vi "Const-BaudDetect-Array.vi"() -> (0 "DetectArray":cluster{"T0":u8, "T1":u8, "br_selfdef":T1}[](array[cluster]) {"T0" format="%08b"; "T1" format="%08b"; "br_selfdef"."PHSEG2" items=["CAN_BIT_1TQ"=1, "CAN_BIT_2TQ"=2, "CAN_BIT_3TQ"=3, "CAN_BIT_4TQ"=4, "CAN_BIT_5TQ"=5, "CAN_BIT_6TQ"=6, "CAN_BIT_7TQ"=7, "CAN_BIT_8TQ"=8]; "br_selfdef"."PHSEG1" items=["CAN_BIT_1TQ"=1, "CAN_BIT_2TQ"=2, "CAN_BIT_3TQ"=3, "CAN_BIT_4TQ"=4, "CAN_BIT_5TQ"=5, "CAN_BIT_6TQ"=6, "CAN_BIT_7TQ"=7, "CAN_BIT_8TQ"=8]; "br_selfdef"."PRSEG" items=["CAN_BIT_1TQ"=1, "CAN_BIT_2TQ"=2, "CAN_BIT_3TQ"=3, "CAN_BIT_4TQ"=4, "CAN_BIT_5TQ"=5, "CAN_BIT_6TQ"=6, "CAN_BIT_7TQ"=7, "CAN_BIT_8TQ"=8]; "br_selfdef"."PHS2_SEL" items=["由相位缓冲段1时间指定", "可编程"]; "br_selfdef"."SAM" items=["采样一次", "采样三次"]; "br_selfdef"."BRP" items=["1"=1, "2"=2, "3"=3, "4"=4, "5"=5, "6"=6, "7"=7, "8"=8, "9"=9, "10"=10, "11"=11, "12"=12, "13"=13, "14"=14, "15"=15, "16"=16, "17"=17, "18"=18, "19"=19, "20"=20, "21"=21, "22"=22, "23"=23, "24"=24, "25"=25, "26"=26, "27"=27, "28"=28, "29"=29, "30"=30, "31"=31, "32"=32, "33"=33, "34"=34, "35"=35, "36"=36, "37"=37, "38"=38, "39"=39, "40"=40, "41"=41, "42"=42, "43"=43, "44"=44, "45"=45, "46"=46, "47"=47, "48"=48, "49"=49, "50"=50, "51"=51, "52"=52, "53"=53, "54"=54, "55"=55, "56"=56, "57"=57, "58"=58, "59"=59, "60"=60, "61"=61, "62"=62, "63"=63, "64"=64]; "br_selfdef"."SJW" items=["1TQ"=1, "2TQ"=2, "3TQ"=3, "4TQ"=4]; "br_selfdef"."SYN(nouse)" items=["CAN_BIT_1TQ"=1]})   [LabVIEW 2011]
uses:
  Baud rate Self Define.ctl
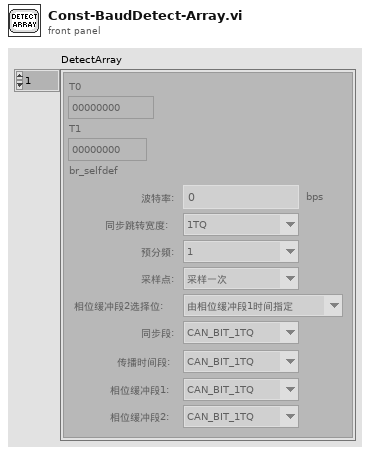
[diagram p1: front panel]
types:
  T1 = typedef "Baud rate Self Define.ctl" = cluster{"BAUD":u32, "SJW":u8, "BRP":u8, "SAM":u8, "PHS2_SEL":u8, "SYN(nouse)":u8, "PRSEG":u8, "PHSEG1":u8, "PHSEG2":u8}
  T2 = cluster{dbl, cluster{"T0":u8, "T1":u8, "br_selfdef":T1}}
  T3 = cluster{dbl, cluster{"T0":u8, "T1":u8, "br_selfdef":T1}}[]
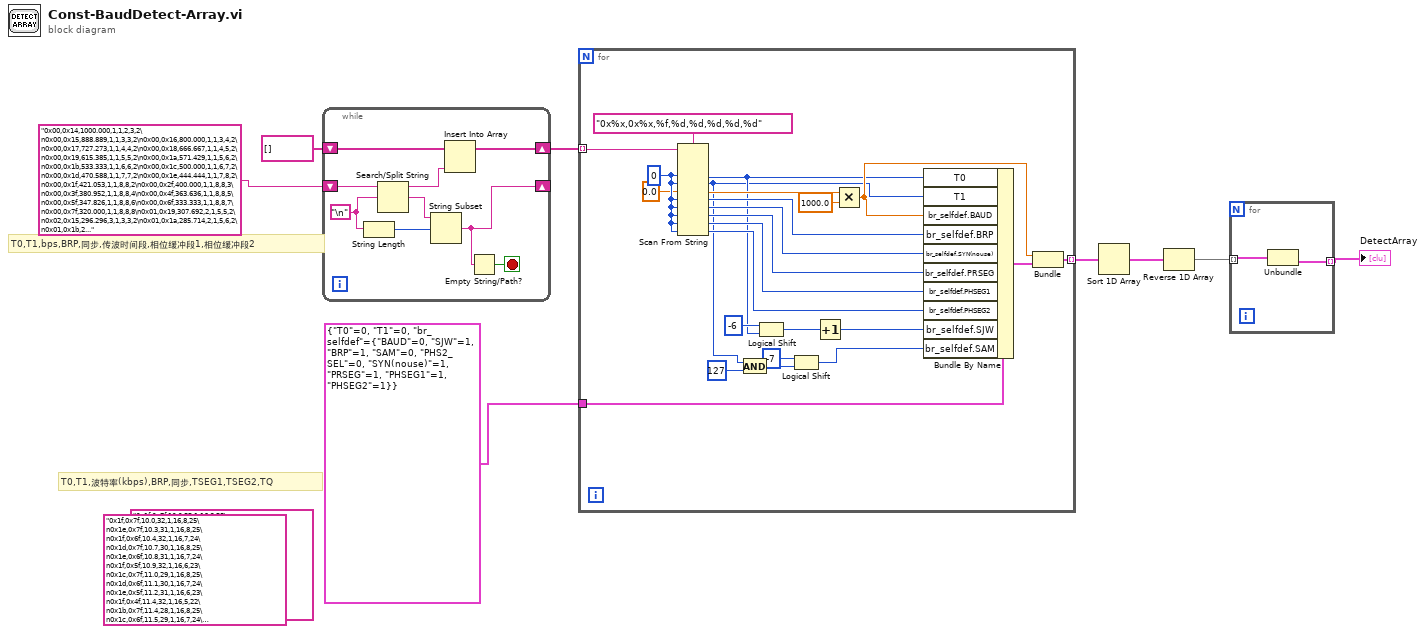
[diagram p0: block diagram]
diagram:
  (unwired) "0x1f,0x7f,10.0,32,1,16,8,25\n0x1e,0x7f,10.3,31,1,16,8,25\n0x1f,0x6f,10.4,32,1,16,7,24\n0x1d,0x7f,10.7,30,1,16,8,25\n0x1e,0x6f,10.8,31,1,16,7,24\n0x1f,0x5f,10.9,32,1,16,6,23\n0x1c,0x7f,11.0,29,1,16,8,25\n0x1d,0x6f,11.1,30,1,16,7,24\n0x1e,0x5f,11.2,31,1,16,6,23\n0x1f,0x4f,11.4,32,1,16,5,22\n0x1b,0x7f,11.4,28,1,16,8,25\n0x1c,0x6f,11.5,29,1,16,7,24\n0x1d,0x5f,11.6,30,1,16,6,23\n0x1e,0x4f,11.7,31,1,16,5,22\n0x1a,0x7f,11.9,27,1,16,8,25\n0x1b,0x6f,11.9,28,1,16,7,24\n0x1c,0x5f,12.0,29,1,16,6,23\n0x1d,0x4f,12.1,30,1,16,5,22\n0x1e,0x3f,12.3,31,1,16,4,21\n0x19,0x7f,12.3,26,1,16,8,25\n0x1a,0x6f,12.3,27,1,16,7,24\n0x1b,0x5f,12.4,28,1,16,6,23\n0x1f,0x2f,12.5,32,1,16,3,20\n0x1c,0x4f,12.5,29,1,16,5,22\n0x1d,0x3f,12.7,30,1,16,4,21\n0x18,0x7f,12.8,25,1,16,8,25\n0x19,0x6f,12.8,26,1,16,7,24\n0x1a,0x5f,12.9,27,1,16,6,23\n0x1e,0x2f,12.9,31,1,16,3,20\n0x1b,0x4f,13.0,28,1,16,5,22\n0x1c,0x3f,13.1,29,1,16,4,21\n0x1f,0x1f,13.2,32,1,16,2,19\n0x17,0x7f,13.3,24,1,16,8,25\n0x19,0x5f,13.4,26,1,16,6,23\n0x1a,0x4f,13.5,27,1,16,5,22\n0x1e,0x1f,13.6,31,1,16,2,19\n0x1b,0x3f,13.6,28,1,16,4,21\n0x1c,0x2f,13.8,29,1,16,3,20\n0x17,0x6f,13.9,24,1,16,7,24\n0x16,0x7f,13.9,23,1,16,8,25\n0x19,0x4f,14.0,26,1,16,5,22\n0x1d,0x1f,14.0,30,1,16,2,19\n0x1a,0x3f,14.1,27,1,16,4,21\n0x1b,0x2f,14.3,28,1,16,3,20\n0x1e,0x1e,14.3,31,1,15,2,18\n0x16,0x6f,14.5,23,1,16,7,24\n0x1c,0x1f,14.5,29,1,16,2,19\n0x15,0x7f,14.5,22,1,16,8,25\n0x19,0x3f,14.7,26,1,16,4,21\n0x1f,0x1d,14.7,32,1,14,2,17\n0x1a,0x2f,14.8,27,1,16,3,20\n0x1b,0x1f,15.0,28,1,16,2,19\n0x16,0x5f,15.1,23,1,16,6,23\n0x15,0x6f,15.2,22,1,16,7,24\n0x1e,0x1d,15.2,31,1,14,2,17\n0x14,0x7f,15.2,21,1,16,8,25\n0x1c,0x1e,15.3,29,1,15,2,18\n0x19,0x2f,15.4,26,1,16,3,20\n0x1a,0x1f,15.6,27,1,16,2,19\n0x1f,0x1c,15.6,32,1,13,2,16\n0x1d,0x1d,15.7,30,1,14,2,17\n0x15,0x5f,15.8,22,1,16,6,23\n0x14,0x6f,15.9,21,1,16,7,24\n0x13,0x7f,16.0,20,1,16,8,25\n0x1e,0x1c,16.1,31,1,13,2,16\n0x19,0x1f,16.2,26,1,16,2,19\n0x1c,0x1d,16.2,29,1,14,2,17\n0x1a,0x1e,16.5,27,1,15,2,18\n0x15,0x4f,16.5,22,1,16,5,22\n0x14,0x5f,16.6,21,1,16,6,23\n0x13,0x6f,16.7,20,1,16,7,24\n0x1b,0x1d,16.8,28,1,14,2,17\n0x12,0x7f,16.8,19,1,16,8,25\n0x19,0x1e,17.1,26,1,15,2,18\n0x1e,0x1b,17.2,31,1,12,2,15\n0x1c,0x1c,17.2,29,1,13,2,16\n0x14,0x4f,17.3,21,1,16,5,22\n0x13,0x5f,17.4,20,1,16,6,23\n0x1a,0x1d,17.4,27,1,14,2,17\n0x12,0x6f,17.5,19,1,16,7,24\n0x11,0x7f,17.8,18,1,16,8,25\n0x1b,0x1c,17.9,28,1,13,2,16\n0x19,0x1d,18.1,26,1,14,2,17\n0x14,0x3f,18.1,21,1,16,4,21\n0x13,0x4f,18.2,20,1,16,5,22\n0x12,0x5f,18.3,19,1,16,6,23\n0x1c,0x1b,18.4,29,1,12,2,15\n0x1e,0x1a,18.4,31,1,11,2,14\n0x11,0x6f,18.5,18,1,16,7,24\n0x10,0x7f,18.8,17,1,16,8,25\n0x13,0x3f,19.0,20,1,16,4,21\n0x12,0x4f,19.1,19,1,16,5,22\n0x19,0x1c,19.2,26,1,13,2,16\n0x11,0x5f,19.3,18,1,16,6,23\n0x10,0x6f,19.6,17,1,16,7,24\n0x1c,0x1a,19.7,29,1,11,2,14\n0x1a,0x1b,19.8,27,1,12,2,15\n0x1e,0x19,19.9,31,1,10,2,13\n0x0f,0x7f,20.0,16,1,16,8,25\n0x12,0x3f,20.1,19,1,16,4,21\n0x11,0x4f,20.2,18,1,16,5,22\n0x1b,0x1a,20.4,28,1,11,2,14\n0x10,0x5f,20.5,17,1,16,6,23\n0x19,0x1b,20.5,26,1,12,2,15\n0x0f,0x6f,20.8,16,1,16,7,24\n0x12,0x2f,21.1,19,1,16,3,20\n0x11,0x3f,21.2,18,1,16,4,21\n0x1c,0x19,21.2,29,1,10,2,13\n0x0e,0x7f,21.3,15,1,16,8,25\n0x10,0x4f,21.4,17,1,16,5,22\n0x1e,0x18,21.5,31,1,9,2,12\n0x0f,0x5f,21.7,16,1,16,6,23\n0x19,0x1a,22.0,26,1,11,2,14\n0x12,0x1f,22.2,19,1,16,2,19\n0x0e,0x6f,22.2,15,1,16,7,24\n0x10,0x3f,22.4,17,1,16,4,21\n0x0f,0x4f,22.7,16,1,16,5,22\n0x1a,0x19,22.8,27,1,10,2,13\n0x0d,0x7f,22.9,14,1,16,8,25\n0x1c,0x18,23.0,29,1,9,2,12\n0x0e,0x5f,23.2,15,1,16,6,23\n0x11,0x1f,23.4,18,1,16,2,19\n0x1e,0x17,23.5,31,1,8,2,11\n0x10,0x2f,23.5,17,1,16,3,20\n0x19,0x19,23.7,26,1,10,2,13\n0x0d,0x6f,23.8,14,1,16,7,24\n0x0e,0x4f,24.2,15,1,16,5,22\n0x0c,0x7f,24.6,13,1,16,8,25\n0x11,0x1e,24.7,18,1,15,2,18\n0x10,0x1f,24.8,17,1,16,2,19\n0x0d,0x5f,24.8,14,1,16,6,23\n0x0f,0x2f,25.0,16,1,16,3,20\n0x1c,0x17,25.1,29,1,8,2,11\n0x0e,0x3f,25.4,15,1,16,4,21\n0x0c,0x6f,25.6,13,1,16,7,24\n0x1e,0x16,25.8,31,1,7,2,10\n0x0d,0x4f,26.0,14,1,16,5,22\n0x10,0x1e,26.1,17,1,15,2,18\n0x0f,0x1f,26.3,16,1,16,2,19\n0x0b,0x7f,26.7,12,1,16,8,25\n0x0c,0x5f,26.8,13,1,16,6,23\n0x1a,0x17,26.9,27,1,8,2,11\n0x0d,0x3f,27.2,14,1,16,4,21\n0x1c,0x16,27.6,29,1,7,2,10\n0x10,0x1d,27.7,17,1,14,2,17\n0x0b,0x6f,27.8,12,1,16,7,24\n0x0c,0x4f,28.0,13,1,16,5,22\n0x0e,0x1f,28.1,15,1,16,2,19\n0x0d,0x2f,28.6,14,1,16,3,20\n0x1e,0x15,28.7,31,1,6,2,9\n0x0b,0x5f,29.0,12,1,16,6,23\n0x0a,0x7f,29.1,11,1,16,8,25\n0x0c,0x3f,29.3,13,1,16,4,21\n0x0f,0x1d,29.4,16,1,14,2,17\n0x0e,0x1e,29.6,15,1,15,2,18\n0x0d,0x1f,30.1,14,1,16,2,19\n0x0a,0x6f,30.3,11,1,16,7,24\n0x1c,0x15,30.7,29,1,6,2,9\n0x0c,0x2f,30.8,13,1,16,3,20\n0x0f,0x1c,31.3,16,1,13,2,16\n0x0e,0x1d,31.4,15,1,14,2,17\n0x0a,0x5f,31.6,11,1,16,6,23\n0x0b,0x3f,31.7,12,1,16,4,21\n0x09,0x7f,32.0,10,1,16,8,25\n0x1e,0x14,32.3,31,1,5,2,8\n0x0c,0x1f,32.4,13,1,16,2,19\n0x1a,0x15,32.9,27,1,6,2,9\n0x0a,0x4f,33.1,11,1,16,5,22\n0x09,0x6f,33.3,10,1,16,7,24\n0x0d,0x1d,33.6,14,1,14,2,17\n0x0c,0x1e,34.2,13,1,15,2,18\n0x1c,0x14,34.5,29,1,5,2,8\n0x0a,0x3f,34.6,11,1,16,4,21\n0x09,0x5f,34.8,10,1,16,6,23\n0x0b,0x1f,35.1,12,1,16,2,19\n0x08,0x7f,35.6,9,1,16,8,25\n0x0d,0x1c,35.7,14,1,13,2,16\n0x0c,0x1d,36.2,13,1,14,2,17\n0x09,0x4f,36.4,10,1,16,5,22\n0x1e,0x13,36.9,31,1,4,2,7\n0x08,0x6f,37.0,9,1,16,7,24\n0x09,0x3f,38.1,10,1,16,4,21\n0x0a,0x1f,38.3,11,1,16,2,19\n0x0c,0x1c,38.5,13,1,13,2,16\n0x08,0x5f,38.6,9,1,16,6,23\n0x0b,0x1d,39.2,12,1,14,2,17\n0x1c,0x13,39.4,29,1,4,2,7\n0x07,0x7f,40.0,8,1,16,8,25\n0x08,0x4f,40.4,9,1,16,5,22\n0x0d,0x1a,40.8,14,1,11,2,14\n0x0c,0x1b,41.0,13,1,12,2,15\n0x07,0x6f,41.7,8,1,16,7,24\n0x09,0x1f,42.1,10,1,16,2,19\n0x08,0x3f,42.3,9,1,16,4,21\n0x0a,0x1d,42.8,11,1,14,2,17\n0x1e,0x12,43.0,31,1,3,2,6\n0x07,0x5f,43.5,8,1,16,6,23\n0x0c,0x1a,44.0,13,1,11,2,14\n0x08,0x2f,44.4,9,1,16,3,20\n0x07,0x4f,45.5,8,1,16,5,22\n0x06,0x7f,45.7,7,1,16,8,25\n0x1c,0x12,46.0,29,1,3,2,6\n0x08,0x1f,46.8,9,1,16,2,19\n0x09,0x1d,47.1,10,1,14,2,17\n0x0c,0x19,47.3,13,1,10,2,13\n0x06,0x6f,47.6,7,1,16,7,24\n0x0a,0x1b,48.5,11,1,12,2,15\n0x08,0x1e,49.4,9,1,15,2,18\n0x06,0x5f,49.7,7,1,16,6,23\n0x07,0x2f,50.0,8,1,16,3,20\n0x0b,0x19,51.3,12,1,10,2,13\n0x1e,0x11,51.6,31,1,2,2,5\n0x06,0x4f,51.9,7,1,16,5,22\n0x08,0x1d,52.3,9,1,14,2,17\n0x07,0x1f,52.6,8,1,16,2,19\n0x05,0x7f,53.3,6,1,16,8,25\n0x06,0x3f,54.4,7,1,16,4,21\n0x1c,0x11,55.2,29,1,2,2,5\n0x05,0x6f,55.6,6,1,16,7,24\n0x0a,0x19,55.9,11,1,10,2,13\n0x06,0x2f,57.1,7,1,16,3,20\n0x05,0x5f,58.0,6,1,16,6,23\n0x07,0x1d,58.8,8,1,14,2,17\n0x08,0x1b,59.3,9,1,12,2,15\n0x06,0x1f,60.2,7,1,16,2,19\n0x05,0x4f,60.6,6,1,16,5,22\n0x09,0x19,61.5,10,1,10,2,13\n0x07,0x1c,62.5,8,1,13,2,16\n0x05,0x3f,63.5,6,1,16,4,21\n0x04,0x7f,64.0,5,1,16,8,25\n0x0a,0x17,66.1,11,1,8,2,11\n0x04,0x6f,66.7,5,1,16,7,24\n0x06,0x1d,67.2,7,1,14,2,17\n0x08,0x19,68.4,9,1,10,2,13\n0x04,0x5f,69.6,5,1,16,6,23\n0x05,0x1f,70.2,6,1,16,2,19\n0x06,0x1c,71.4,7,1,13,2,16\n0x04,0x4f,72.7,5,1,16,5,22\n0x05,0x1e,74.1,6,1,15,2,18\n0x04,0x3f,76.2,5,1,16,4,21\n0x07,0x19,76.9,8,1,10,2,13\n0x05,0x1d,78.4,6,1,14,2,17\n0x03,0x7f,80.0,4,1,16,8,25\n0x08,0x17,80.8,9,1,8,2,11\n0x06,0x1a,81.6,7,1,11,2,14\n0x03,0x6f,83.3,4,1,16,7,24\n0x04,0x1f,84.2,5,1,16,2,19\n0x03,0x5f,87.0,4,1,16,6,23\n0x06,0x19,87.9,7,1,10,2,13\n0x04,0x1e,88.9,5,1,15,2,18\n0x03,0x4f,90.9,4,1,16,5,22\n0x04,0x1d,94.1,5,1,14,2,17\n0x03,0x3f,95.2,4,1,16,4,21\n0x08,0x15,98.8,9,1,6,2,9\n0x03,0x2f,100.0,4,1,16,3,20\n0x05,0x19,102.6,6,1,10,2,13\n0x06,0x17,103.9,7,1,8,2,11\n0x03,0x1f,105.3,4,1,16,2,19\n0x02,0x7f,106.7,3,1,16,8,25\n0x02,0x6f,111.1,3,1,16,7,24\n0x04,0x1a,114.3,5,1,11,2,14\n0x02,0x5f,115.9,3,1,16,6,23\n0x03,0x1d,117.6,4,1,14,2,17\n0x02,0x4f,121.2,3,1,16,5,22\n0x04,0x19,123.1,5,1,10,2,13\n0x03,0x1c,125.0,4,1,13,2,16\n0x02,0x3f,127.0,3,1,16,4,21\n0x02,0x2f,133.3,3,1,16,3,20\n0x02,0x1f,140.4,3,1,16,2,19\n0x03,0x1a,142.9,4,1,11,2,14\n0x04,0x17,145.5,5,1,8,2,11\n0x02,0x1e,148.1,3,1,15,2,18\n0x03,0x19,153.8,4,1,10,2,13\n0x02,0x1d,156.9,3,1,14,2,17\n0x01,0x7f,160.0,2,1,16,8,25\n0x06,0x13,163.3,7,1,4,2,7\n0x01,0x6f,166.7,2,1,16,7,24\n0x01,0x5f,173.9,2,1,16,6,23\n0x02,0x1b,177.8,3,1,12,2,15\n0x01,0x4f,181.8,2,1,16,5,22\n0x01,0x3f,190.5,2,1,16,4,21\n0x01,0x2f,200.0,2,1,16,3,20\n0x02,0x19,205.1,3,1,10,2,13\n0x01,0x1f,210.5,2,1,16,2,19\n0x01,0x1e,222.2,2,1,15,2,18\n0x04,0x13,228.6,5,1,4,2,7\n0x01,0x1d,235.3,2,1,14,2,17\n0x02,0x17,242.4,3,1,8,2,11\n0x01,0x1c,250.0,2,1,13,2,16\n0x01,0x1b,266.7,2,1,12,2,15\n0x01,0x1a,285.7,2,1,11,2,14\n0x02,0x15,296.3,3,1,6,2,9\n0x01,0x19,307.7,2,1,10,2,13\n0x00,0x7f,320.0,1,1,16,8,25\n0x00,0x6f,333.3,1,1,16,7,24\n0x00,0x5f,347.8,1,1,16,6,23\n0x00,0x4f,363.6,1,1,16,5,22\n0x00,0x3f,381.0,1,1,16,4,21\n0x00,0x2f,400.0,1,1,16,3,20\n0x00,0x1f,421.1,1,1,16,2,19\n0x00,0x1e,444.4,1,1,15,2,18\n0x00,0x1d,470.6,1,1,14,2,17\n0x00,0x1c,500.0,1,1,13,2,16\n0x00,0x1b,533.3,1,1,12,2,15\n0x00,0x1a,571.4,1,1,11,2,14\n0x00,0x19,615.4,1,1,10,2,13\n0x00,0x18,666.7,1,1,9,2,12\n0x00,0x17,727.3,1,1,8,2,11\n0x00,0x16,800.0,1,1,7,2,10\n0x00,0x15,888.9,1,1,6,2,9\n0x00,0x14,1000.0,1,1,5,2,8\n0x00,0x13,1142.9,1,1,4,2,7\n0x00,0x12,1333.3,1,1,3,2,6\n0x00,0x11,1600.0,1,1,2,2,5"
  (unwired) "0x1f,0x7f,10.0,32,1,16,8,25\n0x1e,0x7f,10.3,31,1,16,8,25\n0x1f,0x6f,10.4,32,1,16,7,24\n0x1d,0x7f,10.7,30,1,16,8,25\n0x1e,0x6f,10.8,31,1,16,7,24\n0x1f,0x5f,10.9,32,1,16,6,23\n0x1c,0x7f,11.0,29,1,16,8,25\n0x1d,0x6f,11.1,30,1,16,7,24\n0x1e,0x5f,11.2,31,1,16,6,23\n0x1f,0x4f,11.4,32,1,16,5,22\n0x1b,0x7f,11.4,28,1,16,8,25\n0x1c,0x6f,11.5,29,1,16,7,24\n0x1d,0x5f,11.6,30,1,16,6,23\n0x1e,0x4f,11.7,31,1,16,5,22\n0x1a,0x7f,11.9,27,1,16,8,25\n0x1b,0x6f,11.9,28,1,16,7,24\n0x1c,0x5f,12.0,29,1,16,6,23\n0x1d,0x4f,12.1,30,1,16,5,22\n0x1e,0x3f,12.3,31,1,16,4,21\n0x19,0x7f,12.3,26,1,16,8,25\n0x1a,0x6f,12.3,27,1,16,7,24\n0x1b,0x5f,12.4,28,1,16,6,23\n0x1f,0x2f,12.5,32,1,16,3,20\n0x1c,0x4f,12.5,29,1,16,5,22\n0x1d,0x3f,12.7,30,1,16,4,21\n0x18,0x7f,12.8,25,1,16,8,25\n0x19,0x6f,12.8,26,1,16,7,24\n0x1a,0x5f,12.9,27,1,16,6,23\n0x1e,0x2f,12.9,31,1,16,3,20\n0x1b,0x4f,13.0,28,1,16,5,22\n0x1c,0x3f,13.1,29,1,16,4,21\n0x1f,0x1f,13.2,32,1,16,2,19\n0x17,0x7f,13.3,24,1,16,8,25\n0x19,0x5f,13.4,26,1,16,6,23\n0x1a,0x4f,13.5,27,1,16,5,22\n0x1e,0x1f,13.6,31,1,16,2,19\n0x1b,0x3f,13.6,28,1,16,4,21\n0x1c,0x2f,13.8,29,1,16,3,20\n0x17,0x6f,13.9,24,1,16,7,24\n0x16,0x7f,13.9,23,1,16,8,25\n0x19,0x4f,14.0,26,1,16,5,22\n0x1d,0x1f,14.0,30,1,16,2,19\n0x1a,0x3f,14.1,27,1,16,4,21\n0x1b,0x2f,14.3,28,1,16,3,20\n0x1e,0x1e,14.3,31,1,15,2,18\n0x16,0x6f,14.5,23,1,16,7,24\n0x1c,0x1f,14.5,29,1,16,2,19\n0x15,0x7f,14.5,22,1,16,8,25\n0x19,0x3f,14.7,26,1,16,4,21\n0x1f,0x1d,14.7,32,1,14,2,17\n0x1a,0x2f,14.8,27,1,16,3,20\n0x1b,0x1f,15.0,28,1,16,2,19\n0x16,0x5f,15.1,23,1,16,6,23\n0x15,0x6f,15.2,22,1,16,7,24\n0x1e,0x1d,15.2,31,1,14,2,17\n0x14,0x7f,15.2,21,1,16,8,25\n0x1c,0x1e,15.3,29,1,15,2,18\n0x19,0x2f,15.4,26,1,16,3,20\n0x1a,0x1f,15.6,27,1,16,2,19\n0x1f,0x1c,15.6,32,1,13,2,16\n0x1d,0x1d,15.7,30,1,14,2,17\n0x15,0x5f,15.8,22,1,16,6,23\n0x14,0x6f,15.9,21,1,16,7,24\n0x13,0x7f,16.0,20,1,16,8,25\n0x1e,0x1c,16.1,31,1,13,2,16\n0x19,0x1f,16.2,26,1,16,2,19\n0x1c,0x1d,16.2,29,1,14,2,17\n0x1a,0x1e,16.5,27,1,15,2,18\n0x15,0x4f,16.5,22,1,16,5,22\n0x14,0x5f,16.6,21,1,16,6,23\n0x13,0x6f,16.7,20,1,16,7,24\n0x1b,0x1d,16.8,28,1,14,2,17\n0x12,0x7f,16.8,19,1,16,8,25\n0x19,0x1e,17.1,26,1,15,2,18\n0x1e,0x1b,17.2,31,1,12,2,15\n0x1c,0x1c,17.2,29,1,13,2,16\n0x14,0x4f,17.3,21,1,16,5,22\n0x13,0x5f,17.4,20,1,16,6,23\n0x1a,0x1d,17.4,27,1,14,2,17\n0x12,0x6f,17.5,19,1,16,7,24\n0x11,0x7f,17.8,18,1,16,8,25\n0x1b,0x1c,17.9,28,1,13,2,16\n0x19,0x1d,18.1,26,1,14,2,17\n0x14,0x3f,18.1,21,1,16,4,21\n0x13,0x4f,18.2,20,1,16,5,22\n0x12,0x5f,18.3,19,1,16,6,23\n0x1c,0x1b,18.4,29,1,12,2,15\n0x1e,0x1a,18.4,31,1,11,2,14\n0x11,0x6f,18.5,18,1,16,7,24\n0x10,0x7f,18.8,17,1,16,8,25\n0x13,0x3f,19.0,20,1,16,4,21\n0x12,0x4f,19.1,19,1,16,5,22\n0x19,0x1c,19.2,26,1,13,2,16\n0x11,0x5f,19.3,18,1,16,6,23\n0x10,0x6f,19.6,17,1,16,7,24\n0x1c,0x1a,19.7,29,1,11,2,14\n0x1a,0x1b,19.8,27,1,12,2,15\n0x1e,0x19,19.9,31,1,10,2,13\n0x0f,0x7f,20.0,16,1,16,8,25\n0x12,0x3f,20.1,19,1,16,4,21\n0x11,0x4f,20.2,18,1,16,5,22\n0x1b,0x1a,20.4,28,1,11,2,14\n0x10,0x5f,20.5,17,1,16,6,23\n0x19,0x1b,20.5,26,1,12,2,15\n0x0f,0x6f,20.8,16,1,16,7,24\n0x12,0x2f,21.1,19,1,16,3,20\n0x11,0x3f,21.2,18,1,16,4,21\n0x1c,0x19,21.2,29,1,10,2,13\n0x0e,0x7f,21.3,15,1,16,8,25\n0x10,0x4f,21.4,17,1,16,5,22\n0x1e,0x18,21.5,31,1,9,2,12\n0x0f,0x5f,21.7,16,1,16,6,23\n0x19,0x1a,22.0,26,1,11,2,14\n0x12,0x1f,22.2,19,1,16,2,19\n0x0e,0x6f,22.2,15,1,16,7,24\n0x10,0x3f,22.4,17,1,16,4,21\n0x0f,0x4f,22.7,16,1,16,5,22\n0x1a,0x19,22.8,27,1,10,2,13\n0x0d,0x7f,22.9,14,1,16,8,25\n0x1c,0x18,23.0,29,1,9,2,12\n0x0e,0x5f,23.2,15,1,16,6,23\n0x11,0x1f,23.4,18,1,16,2,19\n0x1e,0x17,23.5,31,1,8,2,11\n0x10,0x2f,23.5,17,1,16,3,20\n0x19,0x19,23.7,26,1,10,2,13\n0x0d,0x6f,23.8,14,1,16,7,24\n0x0e,0x4f,24.2,15,1,16,5,22\n0x0c,0x7f,24.6,13,1,16,8,25\n0x11,0x1e,24.7,18,1,15,2,18\n0x10,0x1f,24.8,17,1,16,2,19\n0x0d,0x5f,24.8,14,1,16,6,23\n0x0f,0x2f,25.0,16,1,16,3,20\n0x1c,0x17,25.1,29,1,8,2,11\n0x0e,0x3f,25.4,15,1,16,4,21\n0x0c,0x6f,25.6,13,1,16,7,24\n0x1e,0x16,25.8,31,1,7,2,10\n0x0d,0x4f,26.0,14,1,16,5,22\n0x10,0x1e,26.1,17,1,15,2,18\n0x0f,0x1f,26.3,16,1,16,2,19\n0x0b,0x7f,26.7,12,1,16,8,25\n0x0c,0x5f,26.8,13,1,16,6,23\n0x1a,0x17,26.9,27,1,8,2,11\n0x0d,0x3f,27.2,14,1,16,4,21\n0x1c,0x16,27.6,29,1,7,2,10\n0x10,0x1d,27.7,17,1,14,2,17\n0x0b,0x6f,27.8,12,1,16,7,24\n0x0c,0x4f,28.0,13,1,16,5,22\n0x0e,0x1f,28.1,15,1,16,2,19\n0x0d,0x2f,28.6,14,1,16,3,20\n0x1e,0x15,28.7,31,1,6,2,9\n0x0b,0x5f,29.0,12,1,16,6,23\n0x0a,0x7f,29.1,11,1,16,8,25\n0x0c,0x3f,29.3,13,1,16,4,21\n0x0f,0x1d,29.4,16,1,14,2,17\n0x0e,0x1e,29.6,15,1,15,2,18\n0x0d,0x1f,30.1,14,1,16,2,19\n0x0a,0x6f,30.3,11,1,16,7,24\n0x1c,0x15,30.7,29,1,6,2,9\n0x0c,0x2f,30.8,13,1,16,3,20\n0x0f,0x1c,31.3,16,1,13,2,16\n0x0e,0x1d,31.4,15,1,14,2,17\n0x0a,0x5f,31.6,11,1,16,6,23\n0x0b,0x3f,31.7,12,1,16,4,21\n0x09,0x7f,32.0,10,1,16,8,25\n0x1e,0x14,32.3,31,1,5,2,8\n0x0c,0x1f,32.4,13,1,16,2,19\n0x1a,0x15,32.9,27,1,6,2,9\n0x0a,0x4f,33.1,11,1,16,5,22\n0x09,0x6f,33.3,10,1,16,7,24\n0x0d,0x1d,33.6,14,1,14,2,17\n0x0c,0x1e,34.2,13,1,15,2,18\n0x1c,0x14,34.5,29,1,5,2,8\n0x0a,0x3f,34.6,11,1,16,4,21\n0x09,0x5f,34.8,10,1,16,6,23\n0x0b,0x1f,35.1,12,1,16,2,19\n0x08,0x7f,35.6,9,1,16,8,25\n0x0d,0x1c,35.7,14,1,13,2,16\n0x0c,0x1d,36.2,13,1,14,2,17\n0x09,0x4f,36.4,10,1,16,5,22\n0x1e,0x13,36.9,31,1,4,2,7\n0x08,0x6f,37.0,9,1,16,7,24\n0x09,0x3f,38.1,10,1,16,4,21\n0x0a,0x1f,38.3,11,1,16,2,19\n0x0c,0x1c,38.5,13,1,13,2,16\n0x08,0x5f,38.6,9,1,16,6,23\n0x0b,0x1d,39.2,12,1,14,2,17\n0x1c,0x13,39.4,29,1,4,2,7\n0x07,0x7f,40.0,8,1,16,8,25\n0x08,0x4f,40.4,9,1,16,5,22\n0x0d,0x1a,40.8,14,1,11,2,14\n0x0c,0x1b,41.0,13,1,12,2,15\n0x07,0x6f,41.7,8,1,16,7,24\n0x09,0x1f,42.1,10,1,16,2,19\n0x08,0x3f,42.3,9,1,16,4,21\n0x0a,0x1d,42.8,11,1,14,2,17\n0x1e,0x12,43.0,31,1,3,2,6\n0x07,0x5f,43.5,8,1,16,6,23\n0x0c,0x1a,44.0,13,1,11,2,14\n0x08,0x2f,44.4,9,1,16,3,20\n0x07,0x4f,45.5,8,1,16,5,22\n0x06,0x7f,45.7,7,1,16,8,25\n0x1c,0x12,46.0,29,1,3,2,6\n0x08,0x1f,46.8,9,1,16,2,19\n0x09,0x1d,47.1,10,1,14,2,17\n0x0c,0x19,47.3,13,1,10,2,13\n0x06,0x6f,47.6,7,1,16,7,24\n0x0a,0x1b,48.5,11,1,12,2,15\n0x08,0x1e,49.4,9,1,15,2,18\n0x06,0x5f,49.7,7,1,16,6,23\n0x07,0x2f,50.0,8,1,16,3,20\n0x0b,0x19,51.3,12,1,10,2,13\n0x1e,0x11,51.6,31,1,2,2,5\n0x06,0x4f,51.9,7,1,16,5,22\n0x08,0x1d,52.3,9,1,14,2,17\n0x07,0x1f,52.6,8,1,16,2,19\n0x05,0x7f,53.3,6,1,16,8,25\n0x06,0x3f,54.4,7,1,16,4,21\n0x1c,0x11,55.2,29,1,2,2,5\n0x05,0x6f,55.6,6,1,16,7,24\n0x0a,0x19,55.9,11,1,10,2,13\n0x06,0x2f,57.1,7,1,16,3,20\n0x05,0x5f,58.0,6,1,16,6,23\n0x07,0x1d,58.8,8,1,14,2,17\n0x08,0x1b,59.3,9,1,12,2,15\n0x06,0x1f,60.2,7,1,16,2,19\n0x05,0x4f,60.6,6,1,16,5,22\n0x09,0x19,61.5,10,1,10,2,13\n0x07,0x1c,62.5,8,1,13,2,16\n0x05,0x3f,63.5,6,1,16,4,21\n0x04,0x7f,64.0,5,1,16,8,25\n0x0a,0x17,66.1,11,1,8,2,11\n0x04,0x6f,66.7,5,1,16,7,24\n0x06,0x1d,67.2,7,1,14,2,17\n0x08,0x19,68.4,9,1,10,2,13\n0x04,0x5f,69.6,5,1,16,6,23\n0x05,0x1f,70.2,6,1,16,2,19\n0x06,0x1c,71.4,7,1,13,2,16\n0x04,0x4f,72.7,5,1,16,5,22\n0x05,0x1e,74.1,6,1,15,2,18\n0x04,0x3f,76.2,5,1,16,4,21\n0x07,0x19,76.9,8,1,10,2,13\n0x05,0x1d,78.4,6,1,14,2,17\n0x03,0x7f,80.0,4,1,16,8,25\n0x08,0x17,80.8,9,1,8,2,11\n0x06,0x1a,81.6,7,1,11,2,14\n0x03,0x6f,83.3,4,1,16,7,24\n0x04,0x1f,84.2,5,1,16,2,19\n0x03,0x5f,87.0,4,1,16,6,23\n0x06,0x19,87.9,7,1,10,2,13\n0x04,0x1e,88.9,5,1,15,2,18\n0x03,0x4f,90.9,4,1,16,5,22\n0x04,0x1d,94.1,5,1,14,2,17\n0x03,0x3f,95.2,4,1,16,4,21\n0x08,0x15,98.8,9,1,6,2,9\n0x03,0x2f,100.0,4,1,16,3,20\n0x05,0x19,102.6,6,1,10,2,13\n0x06,0x17,103.9,7,1,8,2,11\n0x03,0x1f,105.3,4,1,16,2,19\n0x02,0x7f,106.7,3,1,16,8,25\n0x02,0x6f,111.1,3,1,16,7,24\n0x04,0x1a,114.3,5,1,11,2,14\n0x02,0x5f,115.9,3,1,16,6,23\n0x03,0x1d,117.6,4,1,14,2,17\n0x02,0x4f,121.2,3,1,16,5,22\n0x04,0x19,123.1,5,1,10,2,13\n0x03,0x1c,125.0,4,1,13,2,16\n0x02,0x3f,127.0,3,1,16,4,21\n0x02,0x2f,133.3,3,1,16,3,20\n0x02,0x1f,140.4,3,1,16,2,19\n0x03,0x1a,142.9,4,1,11,2,14\n0x04,0x17,145.5,5,1,8,2,11\n0x02,0x1e,148.1,3,1,15,2,18\n0x03,0x19,153.8,4,1,10,2,13\n0x02,0x1d,156.9,3,1,14,2,17\n0x01,0x7f,160.0,2,1,16,8,25\n0x06,0x13,163.3,7,1,4,2,7\n0x01,0x6f,166.7,2,1,16,7,24\n0x01,0x5f,173.9,2,1,16,6,23\n0x02,0x1b,177.8,3,1,12,2,15\n0x01,0x4f,181.8,2,1,16,5,22\n0x01,0x3f,190.5,2,1,16,4,21\n0x01,0x2f,200.0,2,1,16,3,20\n0x02,0x19,205.1,3,1,10,2,13\n0x01,0x1f,210.5,2,1,16,2,19\n0x01,0x1e,222.2,2,1,15,2,18\n0x04,0x13,228.6,5,1,4,2,7\n0x01,0x1d,235.3,2,1,14,2,17\n0x02,0x17,242.4,3,1,8,2,11\n0x01,0x1c,250.0,2,1,13,2,16\n0x01,0x1b,266.7,2,1,12,2,15\n0x01,0x1a,285.7,2,1,11,2,14\n0x02,0x15,296.3,3,1,6,2,9\n0x01,0x19,307.7,2,1,10,2,13\n0x00,0x7f,320.0,1,1,16,8,25\n0x00,0x6f,333.3,1,1,16,7,24\n0x00,0x5f,347.8,1,1,16,6,23\n0x00,0x4f,363.6,1,1,16,5,22\n0x00,0x3f,381.0,1,1,16,4,21\n0x00,0x2f,400.0,1,1,16,3,20\n0x00,0x1f,421.1,1,1,16,2,19\n0x00,0x1e,444.4,1,1,15,2,18\n0x00,0x1d,470.6,1,1,14,2,17\n0x00,0x1c,500.0,1,1,13,2,16\n0x00,0x1b,533.3,1,1,12,2,15\n0x00,0x1a,571.4,1,1,11,2,14\n0x00,0x19,615.4,1,1,10,2,13\n0x00,0x18,666.7,1,1,9,2,12\n0x00,0x17,727.3,1,1,8,2,11\n0x00,0x16,800.0,1,1,7,2,10\n0x00,0x15,888.9,1,1,6,2,9\n0x00,0x14,1000.0,1,1,5,2,8\n0x00,0x13,1142.9,1,1,4,2,7\n0x00,0x12,1333.3,1,1,3,2,6\n0x00,0x11,1600.0,1,1,2,2,5"
  # "T0,T1,波特率(kbps),BRP,同步,TSEG1,TSEG2,TQ"
  # "T0,T1,bps,BRP,同步,传波时间段,相位缓冲段1,相位缓冲段2"
  n1 = while {
    shift-right: [w13] -> _
    shift-left: "0x00,0x14,1000.000,1,1,2,3,2\n0x00,0x15,888.889,1,1,3,3,2\n0x00,0x16,800.000,1,1,3,4,2\n0x00,0x17,727.273,1,1,4,4,2\n0x00,0x18,666.667,1,1,4,5,2\n0x00,0x19,615.385,1,1,5,5,2\n0x00,0x1a,571.429,1,1,5,6,2\n0x00,0x1b,533.333,1,1,6,6,2\n0x00,0x1c,500.000,1,1,6,7,2\n0x00,0x1d,470.588,1,1,7,7,2\n0x00,0x1e,444.444,1,1,7,8,2\n0x00,0x1f,421.053,1,1,8,8,2\n0x00,0x2f,400.000,1,1,8,8,3\n0x00,0x3f,380.952,1,1,8,8,4\n0x00,0x4f,363.636,1,1,8,8,5\n0x00,0x5f,347.826,1,1,8,8,6\n0x00,0x6f,333.333,1,1,8,8,7\n0x00,0x7f,320.000,1,1,8,8,8\n0x01,0x19,307.692,2,1,5,5,2\n0x02,0x15,296.296,3,1,3,3,2\n0x01,0x1a,285.714,2,1,5,6,2\n0x01,0x1b,266.667,2,1,6,6,2\n0x01,0x1c,250.000,2,1,6,7,2\n0x02,0x17,242.424,3,1,4,4,2\n0x01,0x1d,235.294,2,1,7,7,2\n0x04,0x13,228.571,5,1,2,2,2\n0x01,0x1e,222.222,2,1,7,8,2\n0x01,0x1f,210.526,2,1,8,8,2\n0x02,0x19,205.128,3,1,5,5,2\n0x01,0x2f,200.000,2,1,8,8,3\n0x01,0x3f,190.476,2,1,8,8,4\n0x01,0x4f,181.818,2,1,8,8,5\n0x02,0x1b,177.778,3,1,6,6,2\n0x01,0x5f,173.913,2,1,8,8,6\n0x01,0x6f,166.667,2,1,8,8,7\n0x06,0x13,163.265,7,1,2,2,2\n0x01,0x7f,160.000,2,1,8,8,8\n0x02,0x1d,156.863,3,1,7,7,2\n0x03,0x19,153.846,4,1,5,5,2\n0x02,0x1e,148.148,3,1,7,8,2\n0x04,0x17,145.455,5,1,4,4,2\n0x03,0x1a,142.857,4,1,5,6,2\n0x02,0x1f,140.351,3,1,8,8,2\n0x02,0x2f,133.333,3,1,8,8,3\n0x02,0x3f,126.984,3,1,8,8,4\n0x03,0x1c,125.000,4,1,6,7,2\n0x04,0x19,123.077,5,1,5,5,2\n0x02,0x4f,121.212,3,1,8,8,5\n0x03,0x1d,117.647,4,1,7,7,2\n0x02,0x5f,115.942,3,1,8,8,6\n0x04,0x1a,114.286,5,1,5,6,2\n0x02,0x6f,111.111,3,1,8,8,7\n0x02,0x7f,106.667,3,1,8,8,8\n0x03,0x1f,105.263,4,1,8,8,2\n0x06,0x17,103.896,7,1,4,4,2\n0x05,0x19,102.564,6,1,5,5,2\n0x03,0x2f,100.000,4,1,8,8,3\n0x08,0x15,98.765,9,1,3,3,2\n0x03,0x3f,95.238,4,1,8,8,4\n0x04,0x1d,94.118,5,1,7,7,2\n0x03,0x4f,90.909,4,1,8,8,5\n0x04,0x1e,88.889,5,1,7,8,2\n0x06,0x19,87.912,7,1,5,5,2\n0x03,0x5f,86.957,4,1,8,8,6\n0x04,0x1f,84.211,5,1,8,8,2\n0x03,0x6f,83.333,4,1,8,8,7\n0x06,0x1a,81.633,7,1,5,6,2\n0x08,0x17,80.808,9,1,4,4,2\n0x03,0x7f,80.000,4,1,8,8,8\n0x05,0x1d,78.431,6,1,7,7,2\n0x07,0x19,76.923,8,1,5,5,2\n0x04,0x3f,76.190,5,1,8,8,4\n0x05,0x1e,74.074,6,1,7,8,2\n0x04,0x4f,72.727,5,1,8,8,5\n0x06,0x1c,71.429,7,1,6,7,2\n0x05,0x1f,70.175,6,1,8,8,2\n0x04,0x5f,69.565,5,1,8,8,6\n0x08,0x19,68.376,9,1,5,5,2\n0x06,0x1d,67.227,7,1,7,7,2\n0x04,0x6f,66.667,5,1,8,8,7\n0x0a,0x17,66.116,11,1,4,4,2\n0x04,0x7f,64.000,5,1,8,8,8\n0x05,0x3f,63.492,6,1,8,8,4\n0x07,0x1c,62.500,8,1,6,7,2\n0x09,0x19,61.538,10,1,5,5,2\n0x05,0x4f,60.606,6,1,8,8,5\n0x06,0x1f,60.150,7,1,8,8,2\n0x08,0x1b,59.259,9,1,6,6,2\n0x07,0x1d,58.824,8,1,7,7,2\n0x05,0x5f,57.971,6,1,8,8,6\n0x06,0x2f,57.143,7,1,8,8,3\n0x0a,0x19,55.944,11,1,5,5,2\n0x05,0x6f,55.556,6,1,8,8,7\n0x1c,0x11,55.172,29,1,1,1,2\n0x06,0x3f,54.422,7,1,8,8,4\n0x05,0x7f,53.333,6,1,8,8,8\n0x07,0x1f,52.632,8,1,8,8,2\n0x08,0x1d,52.288,9,1,7,7,2\n0x06,0x4f,51.948,7,1,8,8,5\n0x1e,0x11,51.613,31,1,1,1,2\n0x0b,0x19,51.282,12,1,5,5,2\n0x07,0x2f,50.000,8,1,8,8,3\n0x06,0x5f,49.689,7,1,8,8,6\n0x08,0x1e,49.383,9,1,7,8,2\n0x0a,0x1b,48.485,11,1,6,6,2\n0x06,0x6f,47.619,7,1,8,8,7\n0x0c,0x19,47.337,13,1,5,5,2\n0x09,0x1d,47.059,10,1,7,7,2\n0x08,0x1f,46.784,9,1,8,8,2\n0x1c,0x12,45.977,29,1,1,2,2\n0x06,0x7f,45.714,7,1,8,8,8\n0x07,0x4f,45.455,8,1,8,8,5\n0x08,0x2f,44.444,9,1,8,8,3\n0x0c,0x1a,43.956,13,1,5,6,2\n0x07,0x5f,43.478,8,1,8,8,6\n0x1e,0x12,43.011,31,1,1,2,2\n0x0a,0x1d,42.781,11,1,7,7,2\n0x08,0x3f,42.328,9,1,8,8,4\n0x09,0x1f,42.105,10,1,8,8,2\n0x07,0x6f,41.667,8,1,8,8,7\n0x0c,0x1b,41.026,13,1,6,6,2\n0x0d,0x1a,40.816,14,1,5,6,2\n0x08,0x4f,40.404,9,1,8,8,5\n0x07,0x7f,40.000,8,1,8,8,8\n0x1c,0x13,39.409,29,1,2,2,2\n0x0b,0x1d,39.216,12,1,7,7,2\n0x08,0x5f,38.647,9,1,8,8,6\n0x0c,0x1c,38.462,13,1,6,7,2\n0x0a,0x1f,38.278,11,1,8,8,2\n0x09,0x3f,38.095,10,1,8,8,4\n0x08,0x6f,37.037,9,1,8,8,7\n0x1e,0x13,36.866,31,1,2,2,2\n0x09,0x4f,36.364,10,1,8,8,5\n0x0c,0x1d,36.199,13,1,7,7,2\n0x0d,0x1c,35.714,14,1,6,7,2\n0x08,0x7f,35.556,9,1,8,8,8\n0x0b,0x1f,35.088,12,1,8,8,2\n0x09,0x5f,34.783,10,1,8,8,6\n0x0a,0x3f,34.632,11,1,8,8,4\n0x1c,0x14,34.483,29,1,2,3,2\n0x0c,0x1e,34.188,13,1,7,8,2\n0x0d,0x1d,33.613,14,1,7,7,2\n0x09,0x6f,33.333,10,1,8,8,7\n0x0a,0x4f,33.058,11,1,8,8,5\n0x1a,0x15,32.922,27,1,3,3,2\n0x0c,0x1f,32.389,13,1,8,8,2\n0x1e,0x14,32.258,31,1,2,3,2\n0x09,0x7f,32.000,10,1,8,8,8\n0x0b,0x3f,31.746,12,1,8,8,4\n0x0a,0x5f,31.621,11,1,8,8,6\n0x0e,0x1d,31.373,15,1,7,7,2\n0x0f,0x1c,31.250,16,1,6,7,2\n0x0c,0x2f,30.769,13,1,8,8,3\n0x1c,0x15,30.651,29,1,3,3,2\n0x0a,0x6f,30.303,11,1,8,8,7\n0x0d,0x1f,30.075,14,1,8,8,2\n0x0e,0x1e,29.630,15,1,7,8,2\n0x0f,0x1d,29.412,16,1,7,7,2\n0x0c,0x3f,29.304,13,1,8,8,4\n0x0a,0x7f,29.091,11,1,8,8,8\n0x0b,0x5f,28.986,12,1,8,8,6\n0x1e,0x15,28.674,31,1,3,3,2\n0x0d,0x2f,28.571,14,1,8,8,3\n0x0e,0x1f,28.070,15,1,8,8,2\n0x0c,0x4f,27.972,13,1,8,8,5\n0x0b,0x6f,27.778,12,1,8,8,7\n0x10,0x1d,27.682,17,1,7,7,2\n0x1c,0x16,27.586,29,1,3,4,2\n0x0d,0x3f,27.211,14,1,8,8,4\n0x1a,0x17,26.936,27,1,4,4,2\n0x0c,0x5f,26.756,13,1,8,8,6\n0x0b,0x7f,26.667,12,1,8,8,8\n0x0f,0x1f,26.316,16,1,8,8,2\n0x10,0x1e,26.144,17,1,7,8,2\n0x0d,0x4f,25.974,14,1,8,8,5\n0x1e,0x16,25.806,31,1,3,4,2\n0x0c,0x6f,25.641,13,1,8,8,7\n0x0e,0x3f,25.397,15,1,8,8,4\n0x1c,0x17,25.078,29,1,4,4,2\n0x0f,0x2f,25.000,16,1,8,8,3\n0x0d,0x5f,24.845,14,1,8,8,6\n0x10,0x1f,24.768,17,1,8,8,2\n0x11,0x1e,24.691,18,1,7,8,2\n0x0c,0x7f,24.615,13,1,8,8,8\n0x0e,0x4f,24.242,15,1,8,8,5\n0x0d,0x6f,23.810,14,1,8,8,7\n0x19,0x19,23.669,26,1,5,5,2\n0x10,0x2f,23.529,17,1,8,8,3\n0x1e,0x17,23.460,31,1,4,4,2\n0x11,0x1f,23.392,18,1,8,8,2\n0x0e,0x5f,23.188,15,1,8,8,6\n0x1c,0x18,22.989,29,1,4,5,2\n0x0d,0x7f,22.857,14,1,8,8,8\n0x1a,0x19,22.792,27,1,5,5,2\n0x0f,0x4f,22.727,16,1,8,8,5\n0x10,0x3f,22.409,17,1,8,8,4\n0x0e,0x6f,22.222,15,1,8,8,7\n0x12,0x1f,22.161,19,1,8,8,2\n0x19,0x1a,21.978,26,1,5,6,2\n0x0f,0x5f,21.739,16,1,8,8,6\n0x1e,0x18,21.505,31,1,4,5,2\n0x10,0x4f,21.390,17,1,8,8,5\n0x0e,0x7f,21.333,15,1,8,8,8\n0x1c,0x19,21.220,29,1,5,5,2\n0x11,0x3f,21.164,18,1,8,8,4\n0x12,0x2f,21.053,19,1,8,8,3\n0x0f,0x6f,20.833,16,1,8,8,7\n0x19,0x1b,20.513,26,1,6,6,2\n0x10,0x5f,20.460,17,1,8,8,6\n0x1b,0x1a,20.408,28,1,5,6,2\n0x11,0x4f,20.202,18,1,8,8,5\n0x12,0x3f,20.050,19,1,8,8,4\n0x0f,0x7f,20.000,16,1,8,8,8\n0x1e,0x19,19.851,31,1,5,5,2\n0x1a,0x1b,19.753,27,1,6,6,2\n0x1c,0x1a,19.704,29,1,5,6,2\n0x10,0x6f,19.608,17,1,8,8,7\n0x11,0x5f,19.324,18,1,8,8,6\n0x19,0x1c,19.231,26,1,6,7,2\n0x12,0x4f,19.139,19,1,8,8,5\n0x13,0x3f,19.048,20,1,8,8,4\n0x10,0x7f,18.824,17,1,8,8,8\n0x11,0x6f,18.519,18,1,8,8,7\n0x1e,0x1a,18.433,31,1,5,6,2\n0x1c,0x1b,18.391,29,1,6,6,2\n0x12,0x5f,18.307,19,1,8,8,6\n0x13,0x4f,18.182,20,1,8,8,5\n0x14,0x3f,18.141,21,1,8,8,4\n0x19,0x1d,18.100,26,1,7,7,2\n0x1b,0x1c,17.857,28,1,6,7,2\n0x11,0x7f,17.778,18,1,8,8,8\n0x12,0x6f,17.544,19,1,8,8,7\n0x1a,0x1d,17.429,27,1,7,7,2\n0x13,0x5f,17.391,20,1,8,8,6\n0x14,0x4f,17.316,21,1,8,8,5\n0x1c,0x1c,17.241,29,1,6,7,2\n0x1e,0x1b,17.204,31,1,6,6,2\n0x19,0x1e,17.094,26,1,7,8,2\n0x12,0x7f,16.842,19,1,8,8,8\n0x1b,0x1d,16.807,28,1,7,7,2\n0x13,0x6f,16.667,20,1,8,8,7\n0x14,0x5f,16.563,21,1,8,8,6\n0x15,0x4f,16.529,22,1,8,8,5\n0x1a,0x1e,16.461,27,1,7,8,2\n0x1c,0x1d,16.227,29,1,7,7,2\n0x19,0x1f,16.194,26,1,8,8,2\n0x1e,0x1c,16.129,31,1,6,7,2\n0x13,0x7f,16.000,20,1,8,8,8\n0x14,0x6f,15.873,21,1,8,8,7\n0x15,0x5f,15.810,22,1,8,8,6\n0x1d,0x1d,15.686,30,1,7,7,2\n0x1f,0x1c,15.625,32,1,6,7,2\n0x1a,0x1f,15.595,27,1,8,8,2\n0x19,0x2f,15.385,26,1,8,8,3\n0x1c,0x1e,15.326,29,1,7,8,2\n0x14,0x7f,15.238,21,1,8,8,8\n0x1e,0x1d,15.180,31,1,7,7,2\n0x15,0x6f,15.152,22,1,8,8,7\n0x16,0x5f,15.123,23,1,8,8,6\n0x1b,0x1f,15.038,28,1,8,8,2\n0x1a,0x2f,14.815,27,1,8,8,3\n0x1f,0x1d,14.706,32,1,7,7,2\n0x19,0x3f,14.652,26,1,8,8,4\n0x15,0x7f,14.545,22,1,8,8,8\n0x1c,0x1f,14.519,29,1,8,8,2\n0x16,0x6f,14.493,23,1,8,8,7\n0x1e,0x1e,14.337,31,1,7,8,2\n0x1b,0x2f,14.286,28,1,8,8,3\n0x1a,0x3f,14.109,27,1,8,8,4\n0x1d,0x1f,14.035,30,1,8,8,2\n0x19,0x4f,13.986,26,1,8,8,5\n0x16,0x7f,13.913,23,1,8,8,8\n0x17,0x6f,13.889,24,1,8,8,7\n0x1c,0x2f,13.793,29,1,8,8,3\n0x1b,0x3f,13.605,28,1,8,8,4\n0x1e,0x1f,13.582,31,1,8,8,2\n0x1a,0x4f,13.468,27,1,8,8,5\n0x19,0x5f,13.378,26,1,8,8,6\n0x17,0x7f,13.333,24,1,8,8,8\n0x1f,0x1f,13.158,32,1,8,8,2\n0x1c,0x3f,13.136,29,1,8,8,4\n0x1b,0x4f,12.987,28,1,8,8,5\n0x1e,0x2f,12.903,31,1,8,8,3\n0x1a,0x5f,12.882,27,1,8,8,6\n0x19,0x6f,12.821,26,1,8,8,7\n0x18,0x7f,12.800,25,1,8,8,8\n0x1d,0x3f,12.698,30,1,8,8,4\n0x1c,0x4f,12.539,29,1,8,8,5\n0x1f,0x2f,12.500,32,1,8,8,3\n0x1b,0x5f,12.422,28,1,8,8,6\n0x1a,0x6f,12.346,27,1,8,8,7\n0x19,0x7f,12.308,26,1,8,8,8\n0x1e,0x3f,12.289,31,1,8,8,4\n0x1d,0x4f,12.121,30,1,8,8,5\n0x1c,0x5f,11.994,29,1,8,8,6\n0x1b,0x6f,11.905,28,1,8,8,7\n0x1a,0x7f,11.852,27,1,8,8,8\n0x1e,0x4f,11.730,31,1,8,8,5\n0x1d,0x5f,11.594,30,1,8,8,6\n0x1c,0x6f,11.494,29,1,8,8,7\n0x1b,0x7f,11.429,28,1,8,8,8\n0x1f,0x4f,11.364,32,1,8,8,5\n0x1e,0x5f,11.220,31,1,8,8,6\n0x1d,0x6f,11.111,30,1,8,8,7\n0x1c,0x7f,11.034,29,1,8,8,8\n0x1f,0x5f,10.870,32,1,8,8,6\n0x1e,0x6f,10.753,31,1,8,8,7\n0x1d,0x7f,10.667,30,1,8,8,8\n0x1f,0x6f,10.417,32,1,8,8,7\n0x1e,0x7f,10.323,31,1,8,8,8\n0x1f,0x7f,10.000,32,1,8,8,8" -> [w17]
    shift-right: [w10] -> w7
    shift-left: string[] [] -> [w9]
    stop <- w12 stop-if-true
    w15 = "\n"
    n2 = String Length(string=w15) -> (length=w14:i32)
    n3 = Search/Split String(string=w17, search string/char (-)=w15) -> (substring before match=w11:string, match + rest of string=w16:string)  [unwired: 1 in, 1 out]
    n4 = String Subset(string=w16, offset (0)=w14) -> (substring=w13:string)  [unwired: 1 in]
    n5 = Insert Into Array(array=w9, new element=w11) -> (w10:string[])  [unwired: 1 in]
    n6 = Empty String/Path?(string/path=w13) -> (empty?=w12:bool)
  }
  n7 = for {
    tunnel: w7 -> [w41] mode=indexing
    tunnel: cluster{"T0":u8, "T1":u8, "br_selfdef":T1} {"T0"=0, "T1"=0, "br_selfdef"={"BAUD"=0, "SJW"=1, "BRP"=1, "SAM"=0, "PHS2_SEL"=0, "SYN(nouse)"=1, "PRSEG"=1, "PHSEG1"=1, "PHSEG2"=1}} -> [w38]
    tunnel: [w20] -> w5 mode=indexing
    w39 = u8 0 ("默认值 1")
    n8 = Scan From String(format string="0x%x,0x%x,%f,%d,%d,%d,%d,%d" ("格式字符串"), input string=w41, default 1=w39, default 2=w39, default 3=0.0 ("默认值 3"), default 4=w39, default 5=w39, default 6=w39, default 7=w39, default 8=w39) -> (output 1=w19:u8, output 2=w18:u8, output 3=w37:dbl, output 4=w35:u8, output 5=w34:u8, output 6=w33:u8, output 7=w32:u8, output 8=w31:u8)  [unwired: 2 in, 3 out]
    n9 = And(x=w18, y=u8 127) -> (x .and. y?=w26:u8)
    n10 = Logical Shift(y=i8 -6, x=w19) -> (x << y=w27:u8)
    n11 = Logical Shift(y=i8 -7, x=w26) -> (x << y=w24:u8)
    n12 = Increment(x=w27) -> (x+1=w23:u8)
    n13 = Multiply(x=w37, y=1000.0) -> (x*y=w21:dbl)
    n14 = Bundle By Name(cluster=w38, "T0"=w19, "T1"=w18, "br_selfdef.BAUD"=w21, "br_selfdef.BRP"=w35, "br_selfdef.SYN(nouse)"=w34, "br_selfdef.PRSEG"=w33, "br_selfdef.PHSEG1"=w32, "br_selfdef.PHSEG2"=w31, "br_selfdef.SJW"=w23, "br_selfdef.SAM"=w24) -> (w22:cluster{"T0":u8, "T1":u8, "br_selfdef":T1})
    n15 = Bundle(w21, w22) -> (w20:T2)  [unwired: 1 in]
  }
  n16 = Sort 1D Array(array=w5) -> (sorted array=w4:T3)
  n17 = Reverse 1D Array(array=w4) -> (reversed array=w1:T3)
  n18 = for {
    tunnel: w1 -> [w43] mode=indexing
    tunnel: [w42] -> w2 mode=indexing
    n19 = Unbundle(w43) -> (w42:cluster{"T0":u8, "T1":u8, "br_selfdef":T1})  [unwired: 1 out]
  }
  "DetectArray" <- w2
